vi "get_status_power.vi"(8 "error in (no error)":errorcluster, 11 "LightSourceMH110125Tsunami in":refnum<class "LightSourceMH110125Tsunami.lvclass">) -> (0 "error out":errorcluster, 2 "output power":dbl[unit], 3 "LightSourceMH110125Tsunami out":refnum<class "LightSourceMH110125Tsunami.lvclass">)   [LabVIEW 2010, in "LightSourceMH110125Tsunami.lvclass"]
uses:
  LightSourceMH110125Tsunami.lvclass
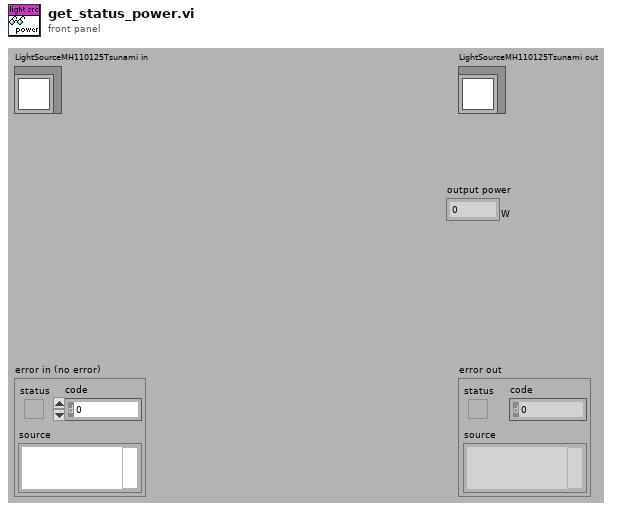
[diagram p1: front panel]
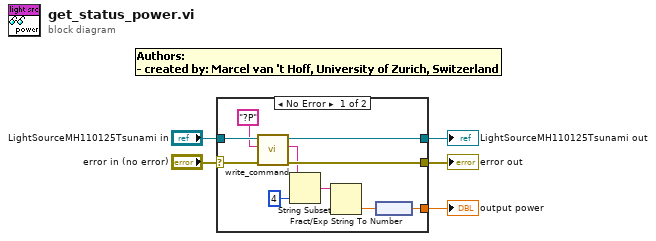
[diagram p0: block diagram]
diagram:
  n1 = case shown="No Error" "error in (no error)" {
    selector: "error in (no error)" -> [w13 w17]
    tunnel: [w12 w17] -> w3
    tunnel: [w14 w16] -> w2
    tunnel: "LightSourceMH110125Tsunami in" -> [w15 w16]
    tunnel: [w7 _] -> w1
    frame No Error {
      n2 = call-dynamic "write_command.vi"("error in (no error)"=w13, "string to write"="?P", "LightSourceMH110125Tsunami in"=w15) -> ("error out"=w12:errorcluster, "read string"=w10:string, "LightSourceMH110125Tsunami out"=w14:refnum<class "LightSourceMH110125Tsunami.lvclass">)  [unwired: 6 in]
      n3 = String Subset(string=w10, length (rest)=4 ("length (rest)")) -> (substring=w9:string)  [unwired: 1 in]
      n4 = Fract/Exp String To Number(string=w9) -> (number=w8:dbl)  [unwired: 3 in, 1 out]
      n5 = node(w8) -> (w7:dbl[unit])
    }
    frame Error {
    }
  }
  "error out" <- w3
  "LightSourceMH110125Tsunami out" <- w2
  "output power" <- w1
